vi "Localization.vi"(1 "Localized Array":string[](array[string])=["Send %s", "%s Msg"], 9 "DNL_Unlocalized Array":string[](array[string])=["Send %s", "%s Msg"], 11 "Unlocalized":string) -> (3 "Localized":string)   [LabVIEW 2016, in "CS++Actor.lvlib" / "CS++Actor.lvclass"]
doc: "Small helper Vi for the localization."
uses:
  CS++Actor.lvclass
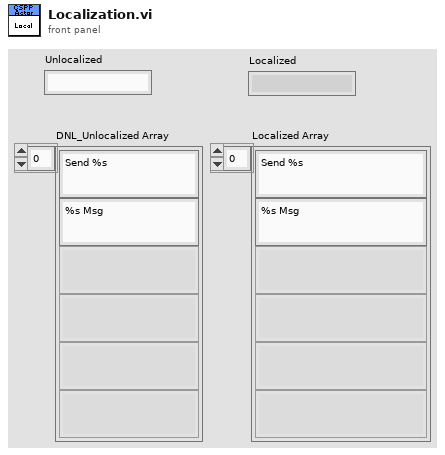
[diagram p1: front panel]
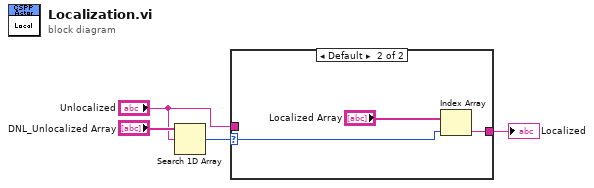
[diagram p0: block diagram]
diagram:
  n1 = Search 1D Array(1D array="DNL_Unlocalized Array", element="Unlocalized") -> (index of element=w2:i32)  [unwired: 1 in]
  n2 = case shown="Default" w2 {
    selector: w2 -> [_ w6]
    tunnel: [w5 w7] -> w3
    tunnel: "Unlocalized" -> [w5 _]
    frame ..-1 {
    }
    frame Default {
      n3 = Index Array(array="Localized Array", index=w6) -> (element=w7:string)
    }
  }
  "Localized" <- w3
